vi "ITC 503 -- read sweep table.vi"(8 "error in":errorcluster, 11 "ITC503 Address":refnum<visa-resource-name>="GPIB0::24::INSTR") -> (0 "error out":errorcluster, 2 "Sweep Table":dbl[][](array[numeric])=[[150.0, 1399.0, 0.0], [20.0, 1399.0, 0.0], [150.0, 1399.0, 0.0], [300.0, 1399.0, 0.0], [295.0, 10.0, 1399.0], [295.0, 10.0, 1399.0]], 3 "ITC503 Address OUT":refnum<visa-resource-name>="GPIB0::24::INSTR")   [LabVIEW 2010]
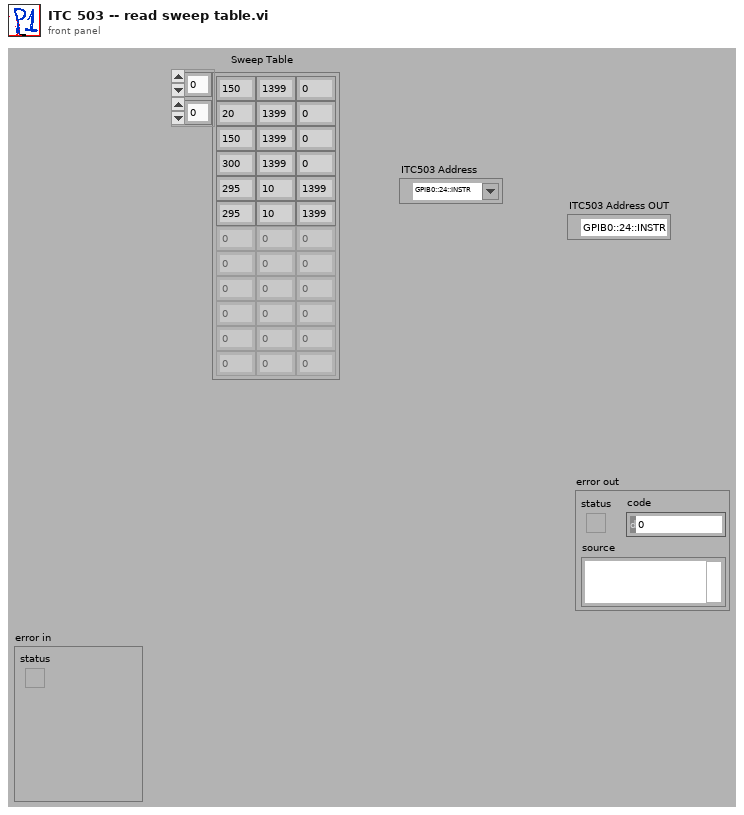
[diagram p1: front panel]
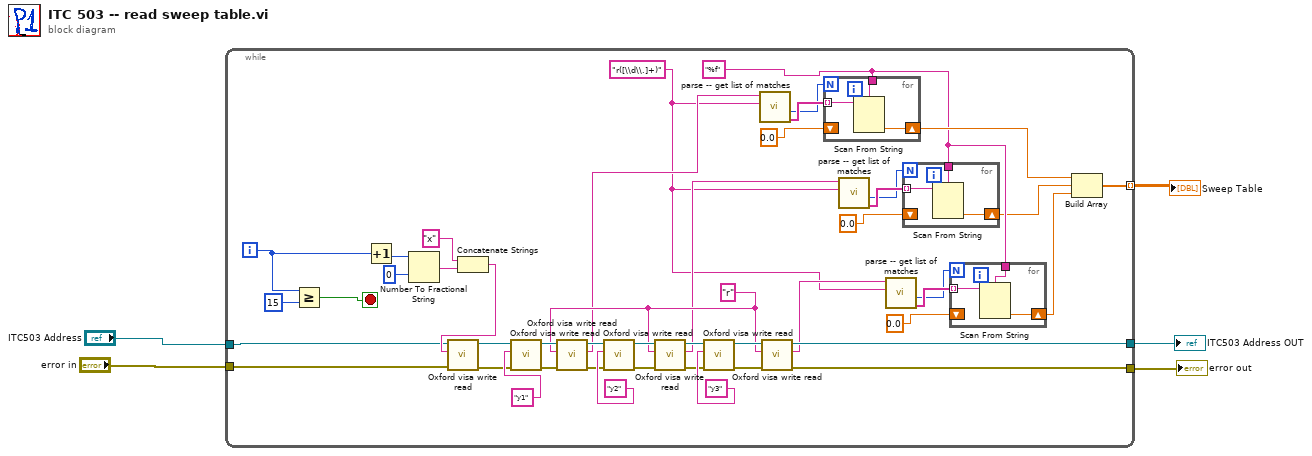
[diagram p0: block diagram]
diagram:
  n1 = while {
    tunnel: "error in" -> [w37]
    tunnel: [w32] -> w4
    tunnel: [w33] -> w3
    tunnel: "ITC503 Address" -> [w28]
    tunnel: [w25] -> w1 mode=indexing
    i -> [w23]
    stop <- w22 stop-if-true
    w9 = "r([\\d\\.]+)" ("format string")
    w8 = "%f" ("format string")
    w27 = "r" ("string")
    n2 = Greater Or Equal?(x=w23, y=15) -> (x >= y?=w22:bool)
    n3 = Increment(x=w23) -> (x+1=w51:i32)
    n4 = Number To Fractional String(number=w51, precision (6)=i16 0) -> (F-format string=w48:string)  [unwired: 2 in]
    n5 = Concatenate Strings("x" ("string"), w48) -> (w47:string)
    n6 = call "Oxford visa write read.vi"("error in (no error)"=w37, "write buffer"=w47, "VISA resource name"=w28) -> ("error out"=w43:errorcluster, "VISA resource name out"=w29:refnum<visa-resource-name>)  [unwired: 6 in, 1 out]
    n7 = call "Oxford visa write read.vi"("error in (no error)"=w43, "write buffer"="y1" ("string"), "VISA resource name"=w29) -> ("error out"=w42:errorcluster, "VISA resource name out"=w30:refnum<visa-resource-name>)  [unwired: 6 in, 1 out]
    n8 = call "Oxford visa write read.vi"("error in (no error)"=w42, "write buffer"=w27, "VISA resource name"=w30) -> ("error out"=w41:errorcluster, "read buffer"=w21:string, "VISA resource name out"=w31:refnum<visa-resource-name>)  [unwired: 6 in]
    n9 = call "Oxford visa write read.vi"("error in (no error)"=w41, "write buffer"="y2" ("string"), "VISA resource name"=w31) -> ("error out"=w40:errorcluster, "VISA resource name out"=w36:refnum<visa-resource-name>)  [unwired: 6 in, 1 out]
    n10 = call "Oxford visa write read.vi"("error in (no error)"=w40, "write buffer"=w27, "VISA resource name"=w36) -> ("error out"=w39:errorcluster, "read buffer"=w10:string, "VISA resource name out"=w35:refnum<visa-resource-name>)  [unwired: 6 in]
    n11 = call "Oxford visa write read.vi"("error in (no error)"=w39, "write buffer"="y3" ("string"), "VISA resource name"=w35) -> ("error out"=w38:errorcluster, "VISA resource name out"=w34:refnum<visa-resource-name>)  [unwired: 6 in, 1 out]
    n12 = call "parse -- get list of matches.vi"("regexp"=w9, "string"=w21) -> ("Array"=w20:string[], "number of free elastic constants"=w19:i32)  [unwired: 7 in, 1 out]
    n13 = call "Oxford visa write read.vi"("error in (no error)"=w38, "write buffer"=w27, "VISA resource name"=w34) -> ("error out"=w32:errorcluster, "read buffer"=w11:string, "VISA resource name out"=w33:refnum<visa-resource-name>)  [unwired: 6 in]
    n14 = for {
      N: w19 -> [_]
      tunnel: w8 -> [w59]
      tunnel: w20 -> [w58] mode=indexing
      shift-right: [w60] -> w26
      shift-left: 0.0 -> [_]
      n15 = Scan From String(format string=w59, input string=w58) -> (output 1=w60:dbl)  [unwired: 3 in, 3 out]
    }
    n16 = call "parse -- get list of matches.vi"("regexp"=w9, "string"=w10) -> ("Array"=w17:string[], "number of free elastic constants"=w16:i32)  [unwired: 7 in, 1 out]
    n17 = call "parse -- get list of matches.vi"("regexp"=w9, "string"=w11) -> ("Array"=w14:string[], "number of free elastic constants"=w13:i32)  [unwired: 7 in, 1 out]
    n18 = for {
      N: w16 -> [_]
      tunnel: w17 -> [w56] mode=indexing
      shift-right: [w57] -> w6
      shift-left: 0.0 -> [_]
      tunnel: w8 -> [w55]
      n19 = Scan From String(format string=w55, input string=w56) -> (output 1=w57:dbl)  [unwired: 3 in, 3 out]
    }
    n20 = for {
      N: w13 -> [_]
      tunnel: w14 -> [w53] mode=indexing
      shift-right: [w54] -> w7
      shift-left: 0.0 -> [_]
      tunnel: w8 -> [w52]
      n21 = Scan From String(format string=w52, input string=w53) -> (output 1=w54:dbl)  [unwired: 3 in, 3 out]
    }
    n22 = Build Array(w26, w6, w7) -> (w25:dbl[])
  }
  "Sweep Table" <- w1
  "error out" <- w4
  "ITC503 Address OUT" <- w3
